vi "StackerController.vi"(0 "HMI to Control":T1={"RightDriveValue"=0.0, "LeftDriveValue"=0.0, "Arm Manual "=0.0, "Stacker Manual "=0.0, "Claw Manual "=0.0, "ClawSlightOpenNumber"=0, "Intake Value "=0.0, "Arm States"=enum."4 Tote", "Claw States"=enum."Claw Manual ", "Intake Man. or Sense"=enum."Sensing", "Stacker in Manual?"=FALSE, "Drop Stack? "=FALSE, "Tusk Up Request"=FALSE, "Tusk Down Request"=FALSE, "Inver. Wheels  In Request"=FALSE, "Inverse. Wheels Out Request "=FALSE, "Get Out of Manual Control"=FALSE, "Exit Score State"=FALSE, "DriveStraight Help?"=FALSE, "Stacker Shut Off No."=0, "Stacker Need Off?"=FALSE, "Collecting?"=FALSE, "Go to Hover"=FALSE, "Stack Clamp Lock "=FALSE, "Stack Clamp Unlock "=FALSE, "Claw Intake Value "=0.0, "Stack Clamp Lock No. "=0, "Steal Can (ruin their day?)"=FALSE, "Retract (have mercy?)"=FALSE, "Can Grab No. "=0, "Wench Value to Control "=0.0}, 1 "SensorInputData":T5, 2 "StackerStates":T6=enum."Hold6", 3 "Disabled?":bool, 4 "Number of Totes":u8) -> (7 "Final Stacker Output":dbl, 8 "Stacker Off?":bool)   [LabVIEW 2014]
uses:
  Typedefs/StackerStates.ctl
  Typedefs/SensorInputData.ctl
  Typedefs/HMI_to_Control.ctl
  Typedefs/Arm States.ctl
  Typedefs/ClawStates.ctl
  Typedefs/IntakeWheelSenseOrManual.ctl
  Gensubs/Bert_or_Ernie.vi
panel:
  out "Power Output Chart":dbl(graph)
  in  "Vt":cluster{"Velocity ":dbl, "Acceleration":dbl}
  out "Stacker Velocity Chart":cluster{"Velocity ":dbl, "Acceleration":dbl}(graph)
  in  "Stacker Ramp Step":dbl=0.02 format="%#_13g"
  in  "permissable stacker error range":dbl=0.1
  out "P,I,D, total output, variable chart":cluster{"P":dbl, "I":dbl, "D":dbl, "P+I+D":dbl}(graph)
  out "Stacker Height, Setpoint, Chart":cluster{"StackerHeight":dbl, "Setpoint":dbl}(graph)
  out "Device has arrived":bool
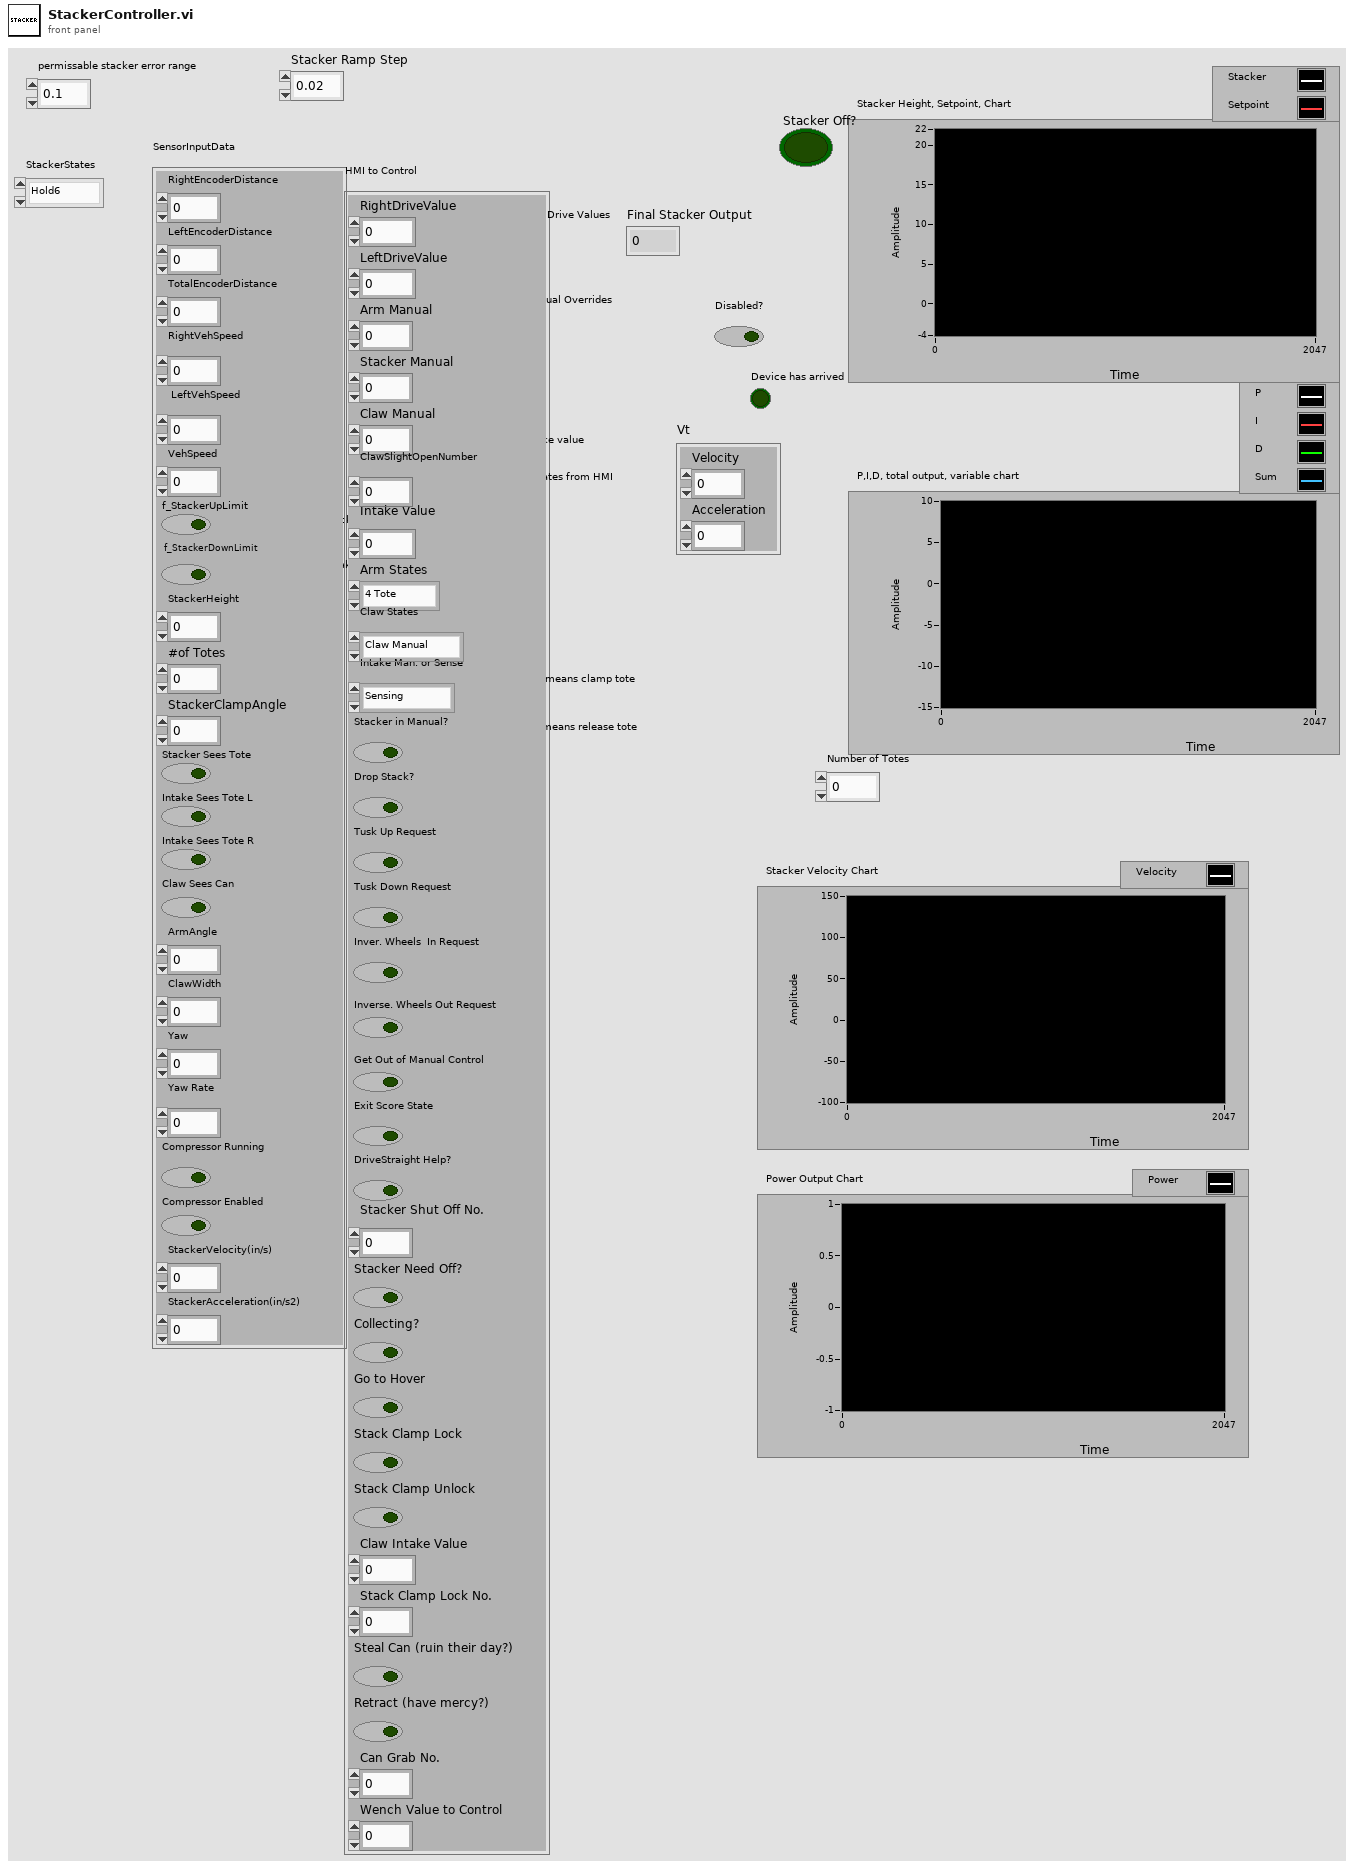
[diagram p1: front panel]
types:
  T1 = typedef "HMI_to_Control.ctl" = cluster{"RightDriveValue":dbl, "LeftDriveValue":dbl, "Arm Manual ":dbl, "Stacker Manual ":dbl, "Claw Manual ":dbl, "ClawSlightOpenNumber":i8, "Intake Value ":sgl, "Arm States":T2, "Claw States":T3, "Intake Man. or Sense":T4, "Stacker in Manual?":bool, "Drop Stack? ":bool, "Tusk Up Request":bool, "Tusk Down Request":bool, "Inver. Wheels  In Request":bool, "Inverse. Wheels Out Request ":bool, "Get Out of Manual Control":bool, "Exit Score State":bool, "DriveStraight Help?":bool, "Stacker Shut Off No.":i8, "Stacker Need Off?":bool, "Collecting?":bool, "Go to Hover":bool, "Stack Clamp Lock ":bool, "Stack Clamp Unlock ":bool, "Claw Intake Value ":sgl, "Stack Clamp Lock No. ":i8, "Steal Can (ruin their day?)":bool, "Retract (have mercy?)":bool, "Can Grab No. ":i8, "Wench Value to Control ":dbl}
  T2 = typedef "Arm States.ctl" = enum16{"Arm Manual ", "Ground", "Step", "1 Tote", "2 Tote", "3 Tote", "4 Tote", "5 Tote", "6 Tote", "Flip Can Arm", "Grab Can in auto", "Nudge"}
  T3 = typedef "ClawStates.ctl" = enum16{"Claw Manual ", "Claw Open", "Claw Closed", "Claw Slight Open", "Flip Can"}
  T4 = typedef "IntakeWheelSenseOrManual.ctl" = enum16{"Sensing", "Manual "}
  T5 = typedef "SensorInputData.ctl" = cluster{"RightEncoderDistance":dbl, "LeftEncoderDistance":dbl, "TotalEncoderDistance":dbl, "RightVehSpeed":dbl, "LeftVehSpeed":dbl, "VehSpeed":dbl, "f_StackerUpLimit":bool, "f_StackerDownLimit":bool, "StackerHeight":dbl, "#of Totes":u8, "StackerClampAngle":dbl, "Stacker Sees Tote":bool, "Intake Sees Tote L":bool, "Intake Sees Tote R":bool, "Claw Sees Can":bool, "ArmAngle":dbl, "ClawWidth":dbl, "Yaw":dbl, "Yaw Rate":dbl, "Compressor Running":bool, "Compressor Enabled":bool, "StackerVelocity(in/s)":dbl, "StackerAcceleration(in/s2)":dbl}
  T6 = typedef "StackerStates.ctl" = enum16{"Manual ", "Hold", "Hold5", "Hold6", "GetTote", "DropStack", "Hover", "Hover5", "Wait for Up", "DecideHold", "DownTimerPeriod", "Prep Intake for Drop", "Check Arm before 5", "Make Arm ready for 5", "Check Arm before 6", "Make Arm ready for 6", "Delay for 5", "Delay for 6"}
  T7 = cluster{"Stacker_kP":dbl, "Stacker_kI":dbl, "Stacker_kD":dbl}
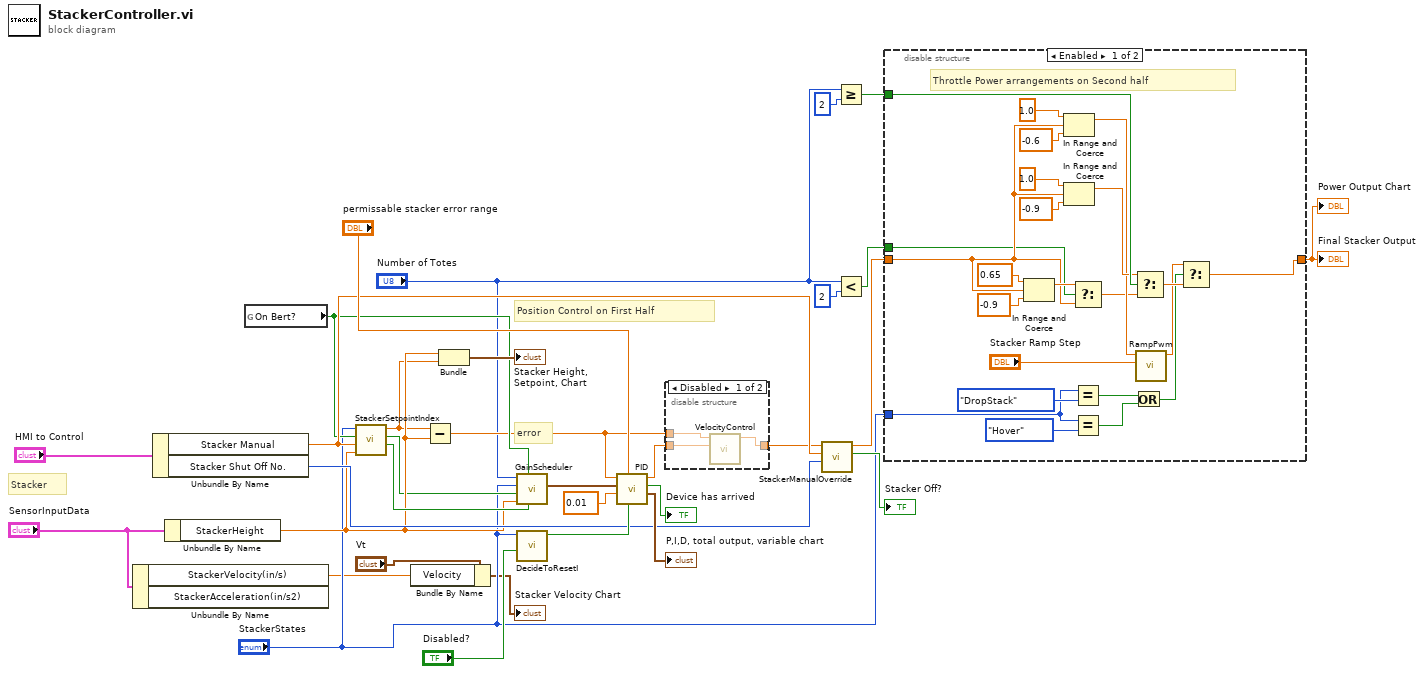
[diagram p0: block diagram]
diagram:
  # "error"
  # "Position Control on First Half"
  # "Stacker"
  n1 = Unbundle By Name("SensorInputData") -> ("StackerVelocity(in/s)"=w10:dbl)  [unwired: 1 out]
  n2 = Unbundle By Name("HMI to Control") -> ("Stacker Manual"=w21:dbl, "Stacker Shut Off No."=w20:i8)
  n3 = Unbundle By Name("SensorInputData") -> ("StackerHeight"=w16:dbl)
  n4 = global read "Bert_or_Ernie.vi" "On Bert?"() -> (w17:bool)
  n5 = call "StackerSetpointIndex.vi"("StackerCurrent"=w16, "Joystick Input"=w21, "On Bert?"=w17, "StackerState"="StackerStates") -> ("Lock Setpoint as Current Height"=w18:bool, "Travel Direction Up"=w15:bool, "Setpoint"=w13:dbl)  [unwired: 5 in]
  n6 = Bundle By Name(cluster="Vt", "Velocity"=w10) -> (→"Stacker Velocity Chart":cluster{"Velocity ":dbl, "Acceleration":dbl})
  n7 = Subtract(x=w13, y=w16) -> (x-y=w6:dbl)
  n8 = Bundle("StackerHeight"=w16, "Setpoint"=w13) -> (→"Stacker Height, Setpoint, Chart":cluster{"StackerHeight":dbl, "Setpoint":dbl})  [unwired: 1 in]
  n9 = call "GainScheduler.vi"("LockSetpoint"=w18, "On Bert?"=w17, "Stacker Height"=w16, "Travel Direction Up"=w15, "StackerState"="StackerStates", "Number of Totes"="Number of Totes") -> ("Stacker Gains Out"=w30:T7)  [unwired: 5 in]
  n10 = call "DecideToResetI.vi"("Disabled?"="Disabled?", "StackerState"="StackerStates") -> ("Reset I"=w31:bool)  [unwired: 9 in]
  n11 = call "PID.vi"("Reset I?"=w31, "permissable error range"="permissable stacker error range", "Loop Period"=0.01, "Gains"=w30, "Error"=w6) -> ("PID Variables"=→"P,I,D, total output, variable chart":cluster{"P":dbl, "I":dbl, "D":dbl, "P+I+D":dbl}, "Device has arrived"=→"Device has arrived":bool, "Output"=w5:dbl)  [unwired: 4 in]
  n12 = disable-structure shown="Disabled" {
    disable-tunnel: w6 -> [w35 _]
    disable-tunnel: w5 -> [w34 w36]
    disable-tunnel: [w33 w36] -> w4
    frame Disabled {
      n13 = call "VelocityControl.vi"("Power from PID"=w34, "Error"=w35) -> ("Final Output"=w33:dbl)  [unwired: 9 in]
    }
    frame Enabled {
    }
  }
  n14 = call "StackerManualOverride.vi"("Shut Off No."=w20, "Stacker Manual"=w21, "Stacker Output"=w4) -> ("Stacker Off?"=→"Stacker Off?":bool, "Final Stacker Output"=w12:dbl)  [unwired: 7 in]
  n15 = Greater Or Equal?(x="Number of Totes", y=2) -> (x >= y?=w22:bool)
  n16 = Less?(x="Number of Totes", y=u8 2) -> (x < y?=w1:bool)
  n17 = disable-structure shown="Enabled" {
    disable-tunnel: w22 -> [w59 _]
    disable-tunnel: "StackerStates" -> [w49 _]
    disable-tunnel: w12 -> [w38 w60]
    disable-tunnel: [w43 w60] -> w7
    disable-tunnel: w1 -> [w37 _]
    frame Enabled {
      # "Throttle Power arrangements on Second half"
      n18 = In Range and Coerce(upper limit=0.65, x=w38, lower limit=-0.9) -> (coerced(x)=w39:dbl)  [unwired: 1 out]
      n19 = In Range and Coerce(upper limit=1.0, x=w38, lower limit=-0.6) -> (coerced(x)=w45:dbl)  [unwired: 1 out]
      n20 = In Range and Coerce(upper limit=1.0, x=w38, lower limit=-0.9) -> (coerced(x)=w56:dbl)  [unwired: 1 out]
      n21 = Select(t=w39, s=w37, f=w38) -> (s? t:f=w40:dbl)
      n22 = Equal?(x=w49, y=StackerStates."DropStack") -> (x = y?=w51:bool)
      n23 = Equal?(x=w49, y=StackerStates."Hover") -> (x = y?=w50:bool)
      n24 = Or(x=w51, y=w50) -> (x .or. y?=w47:bool)
      n25 = Select(t=w56, s=w59, f=w40) -> (s? t:f=w52:dbl)
      n26 = call "RampPwm.vi"("Ramp Step"="Stacker Ramp Step", "Input"=w45) -> ("Output"=w44:dbl)  [unwired: 9 in]
      n27 = Select(t=w44, s=w47, f=w52) -> (s? t:f=w43:dbl)
    }
    frame Disabled {
    }
  }
  "Final Stacker Output" <- w7
  "Power Output Chart" <- w7
